vi "TCP_W.vi"(8 "error in":errorcluster, 9 "timeout ms":i32, 10 "data in":string, 11 "connection ID":refnum<k5>) -> (0 "error IO":errorcluster, 3 "connection ID out":refnum<k5>)   [LabVIEW 2011]
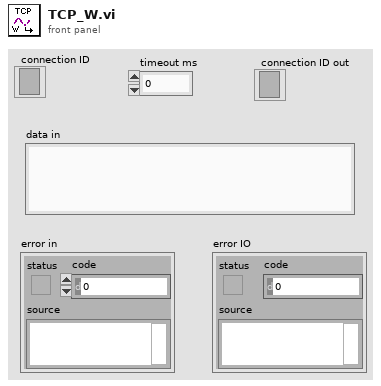
[diagram p1: front panel]
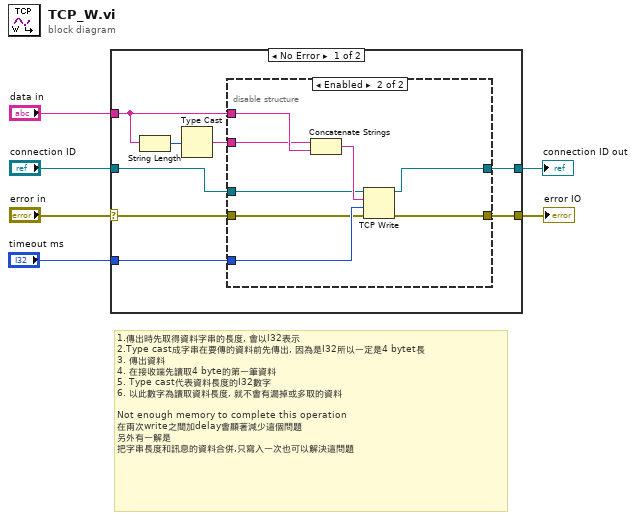
[diagram p0: block diagram]
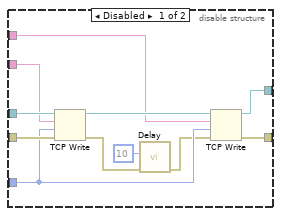
[diagram p2: hidden frame]
diagram:
  # "1.傳出時先取得資料字串的長度, 會以I32表示\n2.Type cast成字串在要傳的資料前先傳出, 因為是I32所以一定是4 bytet長\n3. 傳出資料\n4. 在接收端先讀取4 byte的第一筆資料\n5. Type cast代表資料長度的I32數字\n6. 以此數字為讀取資料長度, 就不會有漏掉或多取的資料\n\nNot enough memory to complete this operation\n在兩次write之間加delay會顯著減少這個問題\n另外有一解是\n把字串長度和訊息的資料合併,只寫入一次也可以解決這問題"
  n1 = case shown="No Error" "error in" {
    selector: "error in" -> [w12 w35]
    tunnel: [w7 w35] -> w3
    tunnel: "connection ID" -> [w13 w34]
    tunnel: "data in" -> [w10 _]
    tunnel: "timeout ms" -> [w9 _]
    tunnel: [w8 w34] -> w1
    frame No Error {
      n2 = String Length(string=w10) -> (length=w14:i32)
      n3 = Type Cast(x=w14) -> (*(type *) &x=w11:string)  [unwired: 1 in]
      n4 = disable-structure shown="Enabled" {
        disable-tunnel: w13 -> [w25 w29]
        disable-tunnel: w12 -> [w23 w26]
        disable-tunnel: w11 -> [w22 w31]
        disable-tunnel: w10 -> [w21 w32]
        disable-tunnel: [w20 w27] -> w7
        disable-tunnel: w9 -> [w19 w30]
        disable-tunnel: [w18 w28] -> w8
        frame Disabled {
          n5 = TCP Write(connection ID=w25, data in=w22, error in (no error)=w23, 9:w19) -> (connection ID out=w24:refnum<k5>, error out=w15:errorcluster)  [unwired: 1 out]
          n6 = call "Delay.vi"("error in"=w15, "delay(ms)"=u32 10) -> ("error out"=w16:errorcluster)  [unwired: 9 in]
          n7 = TCP Write(connection ID=w24, data in=w21, error in (no error)=w16, 9:w19) -> (connection ID out=w18:refnum<k5>, error out=w20:errorcluster)  [unwired: 1 out]
        }
        frame Enabled {
          n8 = Concatenate Strings(w31, w32) -> (w33:string)
          n9 = TCP Write(connection ID=w29, data in=w33, error in (no error)=w26, 9:w30) -> (connection ID out=w28:refnum<k5>, error out=w27:errorcluster)  [unwired: 1 out]
        }
      }
    }
    frame Error {
    }
  }
  "error IO" <- w3
  "connection ID out" <- w1
